vi "find circle corners V2 -- old.vi"(8 "z":cdb[](array[numeric]), 10 "angular distribution in":T2={"histogram - number of  grid points"=100, "theta"=array[300 elements], "histogram"=[]}, 11 "z(center)":cdb=3.141592653589793+0.0i) -> (2 "angular distribution  out":T2={"histogram - number of  grid points"=100, "theta"=array[300 elements], "histogram"=[]}, 3 "circle corners out":T1={"z (-pi/2)"=-1.0311345636926572+0.5736824521422934i, "z(inf)"=-0.5200164984937075+1.0975277942502903i, "z (pi/2)"=-1.0311345636926572+0.5736824521422934i, "z center"=-0.5136528600391839+0.580046090596817i, "z(0)"=-0.5200164984937075+1.0975277942502903i, "radius"=-1.0311345636926572})   [LabVIEW 2010]
uses:
  angular distribution.ctl
  circle corners.ctl
  <vilib>/Analysis/NI_AALBase.lvlib
panel:
  in  "circle corners dummy":T1={"z (-pi/2)"=-1.0311345636926572+0.5736824521422934i, "z(inf)"=-0.5200164984937075+1.0975277942502903i, "z (pi/2)"=-1.0311345636926572+0.5736824521422934i, "z center"=-0.5136528600391839+0.580046090596817i, "z(0)"=-0.5200164984937075+1.0975277942502903i, "radius"=-1.0311345636926572}
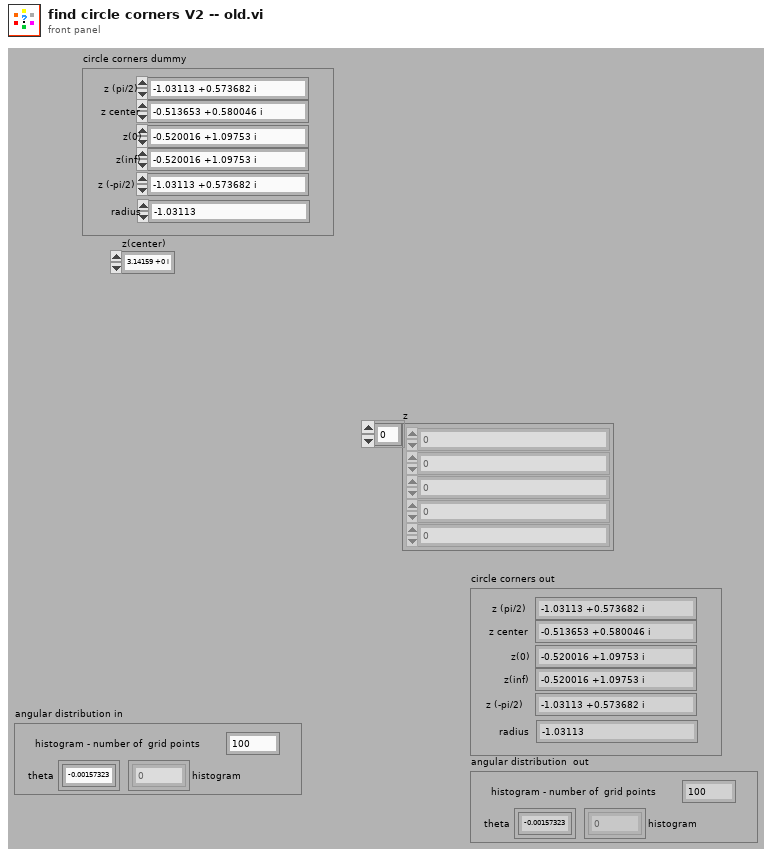
[diagram p1: front panel]
types:
  T1 = typedef "circle corners.ctl" = cluster{"z (-pi/2)":cdb, "z(inf)":cdb, "z (pi/2)":cdb, "z center":cdb, "z(0)":cdb, "radius":dbl}
  T2 = typedef "angular distribution.ctl" = cluster{"histogram - number of  grid points":i32, "theta":dbl[], "histogram":dbl[]}
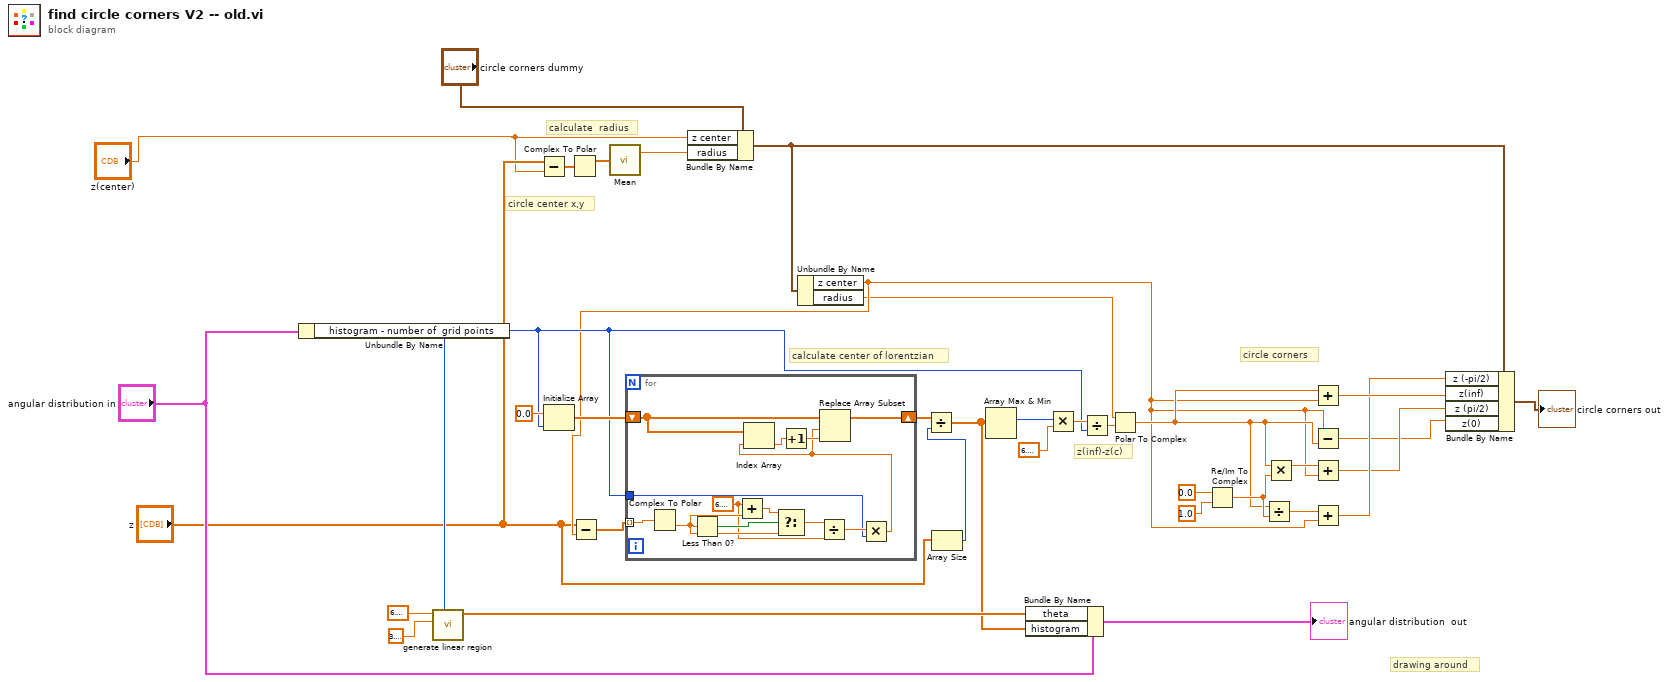
[diagram p0: block diagram]
diagram:
  # "circle center x,y"
  # "calculate  radius"
  # "z(inf)-z(c)"
  # "calculate center of lorentzian"
  # "circle corners"
  # "drawing around"
  n1 = Unbundle By Name("angular distribution in") -> ("histogram - number of  grid points"=w18:i32)
  n2 = call "generate linear region.vi"("number of  grid points"=w18, "center"=3.141592653589793, "delta"=6.283185307179586) -> ("real axis"=w16:dbl[])  [unwired: 8 in]
  n3 = Subtract(x="z", y="z(center)") -> (x-y=w7:cdb[])
  n4 = Initialize Array(0.0 ("element"), w18) -> (w25:dbl[])
  n5 = Complex To Polar(r * e^(i*theta)=w7) -> (r=w6:dbl[])  [unwired: 1 out]
  n6 = call <vilib>:"Mean.vi"("X"=w6) -> ("mean"=w4:dbl)  [unwired: 1 out]
  n7 = Bundle By Name(cluster="circle corners dummy", "z center"="z(center)", "radius"=w4) -> (w1:T1)
  n8 = Unbundle By Name(w1) -> ("z center"=w12:cdb, "radius"=w9:dbl)
  n9 = Subtract(x="z", y=w12) -> (x-y=w13:cdb[])
  n10 = for {
    tunnel: w13 -> [w49] mode=indexing
    shift-right: [w45] -> w24
    shift-left: w25 -> [w46]
    tunnel: w18 -> [w38]
    w40 = 6.283185307179586
    n11 = Complex To Polar(r * e^(i*theta)=w49) -> (theta=w42:dbl)  [unwired: 1 out]
    n12 = Less Than 0?(x=w42) -> (x < 0?=w44:bool)
    n13 = Add(x=w40, y=w42) -> (x+y=w43:dbl)
    n14 = Select(t=w43, s=w44, f=w42) -> (s? t:f=w41:dbl)
    n15 = Divide(x=w41, y=w40) -> (x/y=w39:dbl)
    n16 = Multiply(x=w39, y=w38) -> (x*y=w37:dbl)
    n17 = Index Array(array=w46, index=w37) -> (element=w48:dbl)
    n18 = Increment(x=w48) -> (x+1=w47:dbl)
    n19 = Replace Array Subset(array=w46, new element=w47, index=w37) -> (w45:dbl[])
  }
  n20 = Array Size(array="z") -> (size(s)=w23:i32)
  n21 = Divide(x=w24, y=w23) -> (x/y=w15:dbl[])
  n22 = Array Max & Min(array=w15) -> (max index (indices)=w22:i32)  [unwired: 3 out]
  n23 = Bundle By Name(cluster="angular distribution in", "theta"=w16, "histogram"=w15) -> (→"angular distribution  out":T2)
  n24 = Multiply(x=w22, y=6.283185307179586) -> (x*y=w20:dbl)
  n25 = Divide(x=w20, y=w18) -> (x/y=w19:dbl)
  n26 = Polar To Complex(1:w19, 2:w9) -> (0:w14:cdb)
  n27 = Re/Im To Complex(1:1.0 ("y"), 2:0.0 ("x")) -> (0:w32:cdb)
  n28 = Divide(x=w14, y=w32) -> (x/y=w33:cdb)
  n29 = Multiply(x=w14, y=w32) -> (x*y=w34:cdb)
  n30 = Add(x=w14, y=w12) -> (x+y=w31:cdb)
  n31 = Subtract(x=w12, y=w14) -> (x-y=w8:cdb)
  n32 = Add(x=w34, y=w12) -> (x+y=w29:cdb)
  n33 = Add(x=w33, y=w12) -> (x+y=w30:cdb)
  n34 = Bundle By Name(cluster=w1, "z (-pi/2)"=w30, "z(inf)"=w31, "z (pi/2)"=w29, "z(0)"=w8) -> (→"circle corners out":T1)
